vi "UHR-Fleezers Control (host) -TL - oscillation.vi"(0 "Tab Control":T5(tab)) -> ()   [LabVIEW 2013] (continued)
        n637 = property on="All Signals" class="WFChart (strict)"("Active Plot"=w1031) -> (error out=w1042:errorcluster)  [unwired: 2 in, 1 out]
        n638 = property on="All Signals" class="WFChart (strict)" props=["Plot", "Visible?", "Plot", "Plot Color"](error in=w1042) -> (error out=w1041:errorcluster, "Plot.Visible?"=w1040:bool)  [unwired: 1 in, 2 out]
        n639 = Select(t=FALSE ("Plot.Visible"), s=w1040, f=TRUE ("Plot.Visible")) -> (s? t:f=w1035:bool)
        n640 = property on="All Signals" class="WFChart (strict)"(error in=w1041, "Plot.Visible?"=w1035) -> (error out=w1037:errorcluster)  [unwired: 1 in, 1 out]
        n641 = property on="All Signals" class="WFChart (strict)"(error in=w1037) -> (error out=w1032:errorcluster, "Plot.Plot Color"=w1036:u32)  [unwired: 1 in, 1 out]
        n642 = property on="Signals to Plot" class="LstBox (strict)"(error in=w1032, "Active Row"=w1031) -> (error out=w1030:errorcluster)  [unwired: 1 in, 1 out]
        n643 = Select(t=w1036, s=w1035, f=u32 0) -> (s? t:f=w1033:u32)
        n644 = property on="Signals to Plot" class="LstBox (strict)"(error in=w1030, "CellFontColor"=w1033, "SelColor"=w1029, "CellBG"=w1029, "CellFontSize"=u32 20 ("Active Row:Cell Font:Size"), "CellFontBold"=TRUE ("Active Row:Cell Font:Bold")) -> ()  [unwired: 1 in, 2 out]
      }
      event "BD 1 Frequency 1 (MHz)", "BD 1 Frequency 2 (MHz)", "BD 1 Frequency 3 (MHz)", "BD 2 Frequency 1 (MHz)", "BD 2 Frequency 2 (MHz)", "BD 2 Frequency 3 (MHz)", "Trap Delta (MHz)": Value Change {
        # "anytime one of the frequencies is changed, write it to the RF board UNLESS Set 2 is being oscillated. The oscillation\nscript writes the frequencies to the RF board."
        n645 = event-data() -> ("CtlRef"=w1045:refnum<vi>)  [unwired: 6 out]
        n646 = control-ref of="Trap Delta (MHz)"() -> (w1044:refnum<vi>)
        n647 = Equal?(x=w1044, y=w1045) -> (x = y?=w1043:bool)
        n648 = case shown="False" "Oscillate Traps" {
          tunnel: w1048 -> [w1071 _]
          tunnel: [w1070 w1074] -> w1047
          tunnel: w1046 -> [w1069 w1074]
          tunnel: w1043 -> [w1056 _]
          frame False {
            w1050 = 80
            n649 = local read "BD 1 Frequency 2 (MHz)"() -> (w1058:dbl)
            n650 = Divide(x="Trap Delta (MHz)", y=2) -> (x/y=w1052:dbl)
            n651 = Subtract(x=w1050, y=w1052) -> (x-y=w1051:dbl)
            n652 = local write "BD 1 Frequency 1 (MHz)"(w1051) -> ()
            n653 = Add(x=w1050, y=w1052) -> (x+y=w1057:dbl)
            n654 = Select(t=w1057, s=w1056, f=w1058) -> (s? t:f=w1055:dbl)
            n655 = local read "Y RF Frequency Limits (MHz)"() -> (w1059:T16)
            n656 = local read "X RF Frequency Limits (MHz)"() -> (w1060:T16)
            n657 = local read "BD 1 Frequency 3 (MHz)"() -> (w1072:dbl)
            n658 = local write "BD 1 Frequency 2 (MHz)"(w1055) -> ()
            n659 = local read "BD 2 Frequency 1 (MHz)"() -> (w1063:dbl)
            n660 = local read "BD 2 Frequency 2 (MHz)"() -> (w1062:dbl)
            n661 = local read "BD 2 Frequency 3 (MHz)"() -> (w1073:dbl)
            n662 = call "set RF board frequency - interlace.vi"("Board 2 Frequency Limits"=w1059, "Board 1 Frequency Limits"=w1060, "error in"=w1069, "FPGA VI Reference In"=w1071, "Board 2 Frequency 3 (MHz)"=w1073, "Board 1 Frequency 3 (MHz)"=w1072, "Board 2 Frequency 2 (MHz)"=w1062, "Board 2 Frequency 1 (MHz)"=w1063, "Board 1 Frequency 2 (MHz)"=w1055, "Board 1 Frequency 1  (MHz)"=w1051) -> ("error out"=w1070:errorcluster)  [unwired: 1 out]
            n663 = Subtract(x=w1063, y=w1062) -> (x-y=w1067:dbl)
            n664 = Subtract(x=w1055, y=w1051) -> (x-y=w1068:dbl)
            n665 = Square(x=w1067) -> (x^2=w1065:dbl)
            n666 = Square(x=w1068) -> (x^2=w1066:dbl)
            n667 = Add(x=w1066, y=w1065) -> (x+y=w1064:dbl)
            n668 = Square Root(x=w1064) -> (sqrt(x)=w1061:dbl)
            n669 = local write "Trap Delta (MHz)"(w1061) -> ()
            n670 = property on="Initial delta (MHz)" class="DigNum (strict)"("Val(Sgnl)"=w1061) -> ()  [unwired: 2 in, 2 out]
          }
          frame True {
          }
        }
      }
      event "Round T1 X": Value Change {
        n671 = event-data() -> ()  [unwired: 7 out]
        n672 = local read "BD 1 Frequency 1 (MHz)"() -> (w1077:dbl)
        n673 = Round To Nearest(number=w1077) -> (nearest integer value=w1076:dbl)
        n674 = property on="BD 1 Frequency 1 (MHz)" class="DigNum (strict)"("Val(Sgnl)"=w1076) -> ()  [unwired: 2 in, 2 out]
      }
      event "Restart RF": Value Change {
        n675 = event-data() -> ()  [unwired: 7 out]
        n676 = xnode "Read/Write Control"("FPGA VI Reference In"=w1115, "error in"=w1110, "FPGA Controls  RF Box"=FALSE) -> ("FPGA VI Reference Out"=w1114:T19, "error out"=w1109:errorcluster)
        n677 = local read "Y RF Amplitude Limits (%)"() -> (w1090:T16)
        n678 = local read "X RF Amplitude Limits (%)"() -> (w1091:T16)
        n679 = local read "X RF Frequency Limits (MHz)"() -> (w1093:T16)
        n680 = local read "Y RF Frequency Limits (MHz)"() -> (w1092:T16)
        n681 = xnode "Read/Write Control"("FPGA VI Reference In"=w1114, "error in"=w1109, "Direct RF Box  Communication"=TRUE) -> ("FPGA VI Reference Out"=w1113:T19, "error out"=w1108:errorcluster)
        n682 = local read "BD 2 Frequency 3 (MHz)"() -> (w1100:dbl)
        n683 = local read "BD 2 Frequency 2 (MHz)"() -> (w1101:dbl)
        n684 = local read "BD 1 Frequency 3 (MHz)"() -> (w1104:dbl)
        n685 = local read "BD 1 Frequency 1 (MHz)"() -> (w1105:dbl)
        n686 = local read "BD 2 Frequency 1 (MHz)"() -> (w1102:dbl)
        n687 = local read "BD 1 Frequency 2 (MHz)"() -> (w1103:dbl)
        n688 = call "Initialize RF boards - interlace 3.vi"("error in"=w1108, "FPGA VI Reference In"=w1113) -> ("error out"=w1107:errorcluster, "FPGA VI Reference Out"=w1112:T19)
        n689 = local read "BD 2 Amplitude 2 (%)"() -> (w1095:dbl)
        n690 = local read "BD 2 Amplitude 1 (%)"() -> (w1096:dbl)
        n691 = local read "BD 2 Amplitude 3 (%)"() -> (w1094:dbl)
        n692 = local read "BD 1 Amplitude 3 (%)"() -> (w1099:dbl)
        n693 = local read "BD 1 Amplitude 1 (%)"() -> (w1098:dbl)
        n694 = local read "BD 1 Amplitude 2 (%)"() -> (w1097:dbl)
        n695 = call "set RF board frequency - interlace.vi"("Board 2 Frequency Limits"=w1092, "Board 1 Frequency Limits"=w1093, "error in"=w1107, "FPGA VI Reference In"=w1112, "Board 2 Frequency 3 (MHz)"=w1100, "Board 1 Frequency 3 (MHz)"=w1104, "Board 2 Frequency 2 (MHz)"=w1101, "Board 2 Frequency 1 (MHz)"=w1102, "Board 1 Frequency 2 (MHz)"=w1103, "Board 1 Frequency 1  (MHz)"=w1105) -> ("error out"=w1106:errorcluster, "FPGA VI Reference Out"=w1111:T19)
        n696 = call "set RF board amplitude - interlace.vi"("Board 2 Amplitude Limits"=w1090, "Board 1 Amplitude Limits"=w1091, "error in"=w1106, "FPGA VI Reference In"=w1111, "Board 2 Amplitude 3 (%)"=w1094, "Board 1 Amplitude 3 (%)"=w1099, "Board 2 Amplitude 2 (%)"=w1095, "Board 2 Amplitude 1 (%)"=w1096, "Board 1 Amplitude 2 (%)"=w1097, "Board 1 Amplitude 1 (%)"=w1098) -> ("error out"=w1083:errorcluster, "FPGA VI Reference Out"=w1087:T19)
        n697 = xnode "Read/Write Control"("FPGA VI Reference In"=w1087, "error in"=w1083, "Direct RF Box  Communication"=FALSE) -> ("FPGA VI Reference Out"=w1086:T19, "error out"=w1085:errorcluster)
        n698 = flat-sequence {
          tunnel: w1085 -> [w1116]
          tunnel: [w1116] -> w1084
          frame #0 {
            n699 = Wait (ms)(milliseconds to wait=u32 50) -> ()  [unwired: 1 out]
          }
        }
        n700 = xnode "Read/Write Control"("FPGA VI Reference In"=w1086, "error in"=w1084, "FPGA Controls  RF Box"=TRUE) -> ("error out"=w1079:errorcluster)  [unwired: 1 out]
        n701 = property on="Restart RF" class="Bool (strict)"(error in=w1079, "Value"=FALSE ("Restart RF")) -> (error out=w1078:errorcluster)  [unwired: 1 in, 1 out]
      }
      event "Round T2 X": Value Change {
        n702 = event-data() -> ()  [unwired: 7 out]
        n703 = local read "BD 1 Frequency 2 (MHz)"() -> (w1119:dbl)
        n704 = Round To Nearest(number=w1119) -> (nearest integer value=w1118:dbl)
        n705 = property on="BD 1 Frequency 2 (MHz)" class="DigNum (strict)"("Val(Sgnl)"=w1118) -> ()  [unwired: 2 in, 2 out]
      }
      event "Stop All": Value Change {
        n706 = event-data() -> ()  [unwired: 7 out]
        n707 = call "hamilton_controller.vi"("action"=T20."DISCONNECT") -> ()  [unwired: 10 in, 1 out]
        n708 = local read "Stop All"() -> (w1122:bool)
      }
      event "Delayed Interlace Start": Value Change {
        n709 = event-data() -> ()  [unwired: 7 out]
        n710 = flat-sequence {
          frame #0 {
            n711 = Multiply(x="Delay to Interlace (s)", y=1000.0) -> (x*y=w1125:dbl)
            n712 = Wait (ms)(milliseconds to wait=w1125) -> ()  [unwired: 1 out]
          }
          frame #1 {
            n713 = property on="Green laser mode" class="RadioBtnsControl (strict)"("Val(Sgnl)"=enum32{"Laser ON", "Laser OFF", "Interlace"}."Interlace" ("Value (Signaling)")) -> ()  [unwired: 2 in, 2 out]
          }
        }
      }
      event "BD 1 Amplitude 1 (%)", "BD 1 Amplitude 2 (%)", "BD 1 Amplitude 3 (%)", "BD 2 Amplitude 1 (%)", "BD 2 Amplitude 2 (%)", "BD 2 Amplitude 3 (%)", "Trap 1 ON", "Trap 2 ON", "Trap 3 ON", "Feedback On/Off", "All FB On/Off": Value Change {
        w1149 = i16 1 ("f")
        n714 = event-data() -> ()  [unwired: 7 out]
        n715 = local write "Trap 1 (ON/OFF)"("Trap 1 ON") -> ()
        n716 = local write "Trap 2 (ON/OFF)"("Trap 2 ON") -> ()
        n717 = Boolean To (0,1)(Boolean="Trap 3 ON") -> (0, 1=w1150:i16)
        n718 = Boolean To (0,1)(Boolean="Trap 1 ON") -> (0, 1=w1151:i16)
        n719 = Boolean To (0,1)(Boolean="Trap 2 ON") -> (0, 1=w1152:i16)
        n720 = Select(t=w1152, s="Trap ON/OFF X or Y Amp?", f=w1149) -> (s? t:f=w1147:i16)
        n721 = Select(t=w1151, s="Trap ON/OFF X or Y Amp?", f=w1149) -> (s? t:f=w1148:i16)
        n722 = Select(t=w1150, s="Trap ON/OFF X or Y Amp?", f=w1149) -> (s? t:f=w1146:i16)
        n723 = Select(t=w1149, s="Trap ON/OFF X or Y Amp?", f=w1152) -> (s? t:f=w1144:i16)
        n724 = Select(t=w1149, s="Trap ON/OFF X or Y Amp?", f=w1151) -> (s? t:f=w1145:i16)
        n725 = Select(t=w1149, s="Trap ON/OFF X or Y Amp?", f=w1150) -> (s? t:f=w1143:i16)
        n726 = And(x="All FB On/Off", y="Feedback On/Off") -> (x .and. y?=w1141:cluster{"Set 1":bool, "Set 2":bool})
        n727 = local read "BD 1 Amplitude 1 (%)"() -> (w1161:dbl)
        n728 = local read "BD 1 Amplitude 2 (%)"() -> (w1160:dbl)
        n729 = local read "BD 1 Amplitude 3 (%)"() -> (w1159:dbl)
        n730 = Unbundle By Name(w1141) -> ("Set 1"=w1136:bool, "Set 2"=w1133:bool)
        n731 = local read "Y RF Amplitude Limits (%)"() -> (w1129:T16)
        n732 = local read "X RF Amplitude Limits (%)"() -> (w1130:T16)
        n733 = local read "BD 2 Amplitude 1 (%)"() -> (w1162:dbl)
        n734 = local read "BD 2 Amplitude 2 (%)"() -> (w1163:dbl)
        n735 = local read "BD 2 Amplitude 3 (%)"() -> (w1164:dbl)
        n736 = And(x="Trap 2 ON", y=w1133) -> (x .and. y?=w1131:bool)
        n737 = And(x="Trap 1 ON", y=w1136) -> (x .and. y?=w1134:bool)
        n738 = Multiply(x=w1148, y=w1161) -> (x*y=w1156:dbl)
        n739 = Multiply(x=w1160, y=w1147) -> (x*y=w1154:dbl)
        n740 = Multiply(x=w1159, y=w1146) -> (x*y=w1155:dbl)
        n741 = Multiply(x=w1162, y=w1145) -> (x*y=w1165:dbl)
        n742 = Multiply(x=w1163, y=w1144) -> (x*y=w1166:dbl)
        n743 = Multiply(x=w1164, y=w1143) -> (x*y=w1167:dbl)
        n744 = call "set RF board amplitude - interlace.vi"("Board 2 Amplitude Limits"=w1129, "Board 1 Amplitude Limits"=w1130, "error in"=w1157, "FPGA VI Reference In"=w1158, "Board 2 Amplitude 3 (%)"=w1167, "Board 1 Amplitude 3 (%)"=w1155, "Board 2 Amplitude 2 (%)"=w1166, "Board 2 Amplitude 1 (%)"=w1165, "Board 1 Amplitude 2 (%)"=w1154, "Board 1 Amplitude 1 (%)"=w1156) -> ("error out"=w1138:errorcluster, "FPGA VI Reference Out"=w1139:T19)
        n745 = xnode "Read/Write Control"("FPGA VI Reference In"=w1139, "error in"=w1138, "FB On/Off Set 1"=w1134, "FB On/Off Set 2"=w1131) -> ("error out"=w1137:errorcluster)  [unwired: 1 out]
      }
      event "Load parameters": Value Change {
        n746 = event-data() -> ()  [unwired: 7 out]
        n747 = property on="Saved AOD Raster Scan Parameter Sets" class="Arr (strict)"() -> ("Index Values"=w1178:u32[])  [unwired: 2 in, 2 out]
        n748 = Index Array(array=w1178, index=0) -> (element=w1175:u32)
        n749 = local write "Load parameters"(FALSE ("Load parameters")) -> ()
        n750 = Index Array(array="Saved AOD Raster Scan Parameter Sets", index=w1175) -> (element=w1174:T30)
        n751 = Unbundle By Name(w1174) -> ("Scan Range AOD (nm) 2"=w1173:dbl, "Step Size AOD (nm) 2"=w1172:dbl, "Scan Speed AOD (nm/s) 2"=w1171:dbl, "Number of scans (AOD) 2"=w1170:u16)
        n752 = flat-sequence {
          tunnel: w1173 -> [w1181]
          tunnel: w1172 -> [w1180]
          tunnel: w1171 -> [w1179]
          tunnel: w1170 -> [w1182]
          frame #0 {
            n753 = local write "Scan Speed (nm/s)"(w1179) -> ()
            n754 = local write "Scan Range (nm)"(w1181) -> ()
            n755 = local write "Step Size (nm)"(w1180) -> ()
          }
          frame #1 {
            n756 = property on="Number of F/B Scans (AOD)" class="DigNum (strict)"("Val(Sgnl)"=w1182) -> ()  [unwired: 2 in, 2 out]
          }
        }
      }
      event "Trap 1 (ON/OFF)", "Trap 2 (ON/OFF)": Value Change {
        n757 = event-data() -> ()  [unwired: 7 out]
        n758 = property on="Trap 2 ON" class="Bool (strict)"("Val(Sgnl)"="Trap 2 (ON/OFF)") -> ()  [unwired: 2 in, 2 out]
        n759 = property on="Trap 1 ON" class="Bool (strict)"("Val(Sgnl)"="Trap 1 (ON/OFF)") -> ()  [unwired: 2 in, 2 out]
      }
      event "DIO count 1 (ticks)", "DIO count 2 (ticks)", "DIO count 3 (ticks)", "Interlace", "Number Interlace Sets", "Not-Interlacing Set": Value Change {
        n760 = event-data() -> ()  [unwired: 7 out]
        n761 = local read "DIO count 3 (ticks)"() -> (w1195:u32)
        n762 = local read "DIO count 1 (ticks)"() -> (w1197:u32)
        n763 = local read "DIO count 2 (ticks)"() -> (w1196:u32)
        n764 = To Unsigned Byte Integer(number="Not-Interlacing Set") -> (unsigned 8bit integer=w1186:u8)
        n765 = Add(x=w1186, y=u8 1) -> (x+y=w1190:u8)
        n766 = xnode "Read/Write Control"("FPGA VI Reference In"=w1201, "error in"=w1199, "DIO count 1 (ticks)"=w1197, "DIO count 2 (ticks)"=w1196, "DIO count 3 (ticks)"=w1195, "Interlace ON/OFF"="Interlace", "Number Interlace Cycles"="Number Interlace Sets", "Interlace Off Parameters"=w1190) -> ("error out"=w1200:errorcluster)  [unwired: 1 out]
        n767 = Build Array(w1197, w1196, w1195) -> (w1188:u32[])
        n768 = Split 1D Array(array=w1188, index="Number Interlace Sets") -> (first subarray=w1198:u32[])  [unwired: 1 out]
        n769 = Index Array(array=w1188, index=w1186) -> (element=w1187:u32)
        n770 = Add Array Elements(numeric array=w1198) -> (sum=w1192:u32)
        n771 = Select(t=w1192, s="Interlace", f=w1187) -> (s? t:f=→"Total Counts (ticks)":u32)
      }
      event "Reset Feedback": Value Change {
        n772 = event-data() -> ()  [unwired: 7 out]
        n773 = Unbundle By Name("Reset Feedback") -> ("Set 1"=w1205:bool, "Set 2"=w1204:bool)
        n774 = xnode "Read/Write Control"("FPGA VI Reference In"=w1207, "error in"=w1202, "FB Reset Set 1"=w1205, "FB Reset Set 2"=w1204) -> ("error out"=w1203:errorcluster)  [unwired: 1 out]
      }
      event "PID Gains": Value Change {
        n775 = event-data() -> ()  [unwired: 7 out]
        n776 = Unbundle By Name("PID Gains") -> ("Set 1"=w1211:T14, "Set 2"=w1210:T14)
        n777 = xnode "Read/Write Control"("FPGA VI Reference In"=w1212, "error in"=w1208, "FB Gains Set 1"=w1211, "FB Gains Set 2"=w1210) -> ("error out"=w1209:errorcluster)  [unwired: 1 out]
      }
      event "AI2 to Setpoint", "Trap Intensity\nSetpoints (V)": Value Change {
        n778 = event-data() -> ()  [unwired: 7 out]
        n779 = xnode "Read/Write Control"("FPGA VI Reference In"=w1218, "error in"=w1214) -> ("FPGA VI Reference Out"=w1217:T19, "error out"=w1216:errorcluster, "AI2 Y Sum Set 1"=w1225:i16, "AI2 Y Sum Set 2"=w1224:i16)
        n780 = Cluster To Array(cluster="AI2 to Setpoint") -> (array=w1228:bool[])
        n781 = local read "AI2 (V)"() -> (w1226:cluster{"Set 1":dbl, "Set 2":dbl})
        n782 = Or Array Elements(Boolean array=w1228) -> (logical OR=w1229:bool)
        n783 = Bundle By Name(cluster=w1226, "Set 1"=w1225, "Set 2"=w1224) -> (w1223:cluster{"Set 1":dbl, "Set 2":dbl})
        n784 = Divide(x=w1223, y=3276.7) -> (x/y=w1222:cluster{"Set 1":dbl, "Set 2":dbl})
        "AI2 (V)" <- w1222
        n785 = case shown="True" w1229 {
          tunnel: [w1232 w1249] -> w1221
          tunnel: "AI2 to Setpoint" -> [_ w1245]
          tunnel: "Trap Intensity\nSetpoints (V)" -> [w1233 w1248]
          tunnel: w1222 -> [_ w1242]
          frame False {
            n786 = Multiply(x=3276.7, y=w1233) -> (x*y=w1234:cluster{"Set 1":dbl, "Set 2":dbl})
            n787 = To Word Integer(number=w1234) -> (16bit integer=w1232:cluster{"Set 1":i16, "Set 2":i16})
          }
          frame True {
            n788 = Unbundle By Name(w1242) -> ("Set 1"=w1241:dbl, "Set 2"=w1240:dbl)
            n789 = Unbundle By Name(w1248) -> ("Set 1"=w1247:dbl, "Set 2"=w1246:dbl)
            n790 = Unbundle By Name(w1245) -> ("Set 1"=w1244:bool, "Set 2"=w1243:bool)
            n791 = Select(t=w1241, s=w1244, f=w1247) -> (s? t:f=w1239:dbl)
            n792 = Select(t=w1240, s=w1243, f=w1246) -> (s? t:f=w1238:dbl)
            n793 = Bundle By Name(cluster=w1248, "Set 1"=w1239, "Set 2"=w1238) -> (w1236:cluster{"Set 1":dbl, "Set 2":dbl})
            n794 = local write "Trap Intensity\nSetpoints (V)"(w1236) -> ()
            n795 = Multiply(x=3276.7, y=w1236) -> (x*y=w1237:cluster{"Set 1":dbl, "Set 2":dbl})
            n796 = To Word Integer(number=w1237) -> (16bit integer=w1249:cluster{"Set 1":i16, "Set 2":i16})
          }
        }
        n797 = Unbundle By Name(w1221) -> ("Set 1"=w1220:i16, "Set 2"=w1219:i16)
        n798 = xnode "Read/Write Control"("FPGA VI Reference In"=w1217, "error in"=w1216, "FB Setpoint Set 1"=w1220, "FB Setpoint Set 2"=w1219) -> ("error out"=w1215:errorcluster)  [unwired: 1 out]
      }
      event "Invert GI": Value Change {
        n799 = event-data() -> ()  [unwired: 7 out]
        n800 = xnode "Read/Write Control"("FPGA VI Reference In"=w1254, "error in"=w1252, "Invert GI"="Invert GI", "Invert GI 2"="Invert GI") -> ("error out"=w1253:errorcluster)  [unwired: 1 out]
      }
      event "Green FB Setpoint (mV)", "Green FB Gains", "Green FB On/Off", "Current When FB OFF (%)", "Green int current ON count adj": Value Change {
        n801 = event-data() -> ()  [unwired: 7 out]
        n802 = local read "Green FB Setpoint (mV)"() -> (w1261:dbl)
        n803 = local read "Current When FB OFF (%)"() -> (w1264:dbl)
        n804 = Multiply(x=w1261, y=3.2767) -> (x*y=w1260:dbl)
        n805 = Multiply(x=w1264, y=655.35) -> (x*y=w1265:dbl)
        n806 = To Unsigned Word Integer(number=w1265) -> (unsigned 16bit integer=w1263:u16)
        n807 = local read "Green int current ON count adj"() -> (w1268:u32)
        n808 = local read "Green FB Gains"() -> (w1267:T14)
        n809 = local read "Green Laser ON/Interlacing"() -> (w1258:bool)
        n810 = local read "Green laser mode"() -> (w1257:enum32{"Laser ON", "Laser OFF", "Interlace"})
        n811 = local read "Green FB On/Off"() -> (w1269:bool)
        n812 = Equal?(x=w1257, y=enum32{"Laser ON", "Laser OFF", "Interlace"}."Interlace") -> (x = y?=w1255:bool)
        n813 = Compound Arithmetic op=AND(w1255, w1269, w1258) -> (w1259:bool)
        n814 = xnode "Read/Write Control"("FPGA VI Reference In"=w1272, "error in"=w1271, "Green FB Setpoint"=w1260, "Green FB On/Off"=w1259, "Current Out"=w1263, "Green int current ON count adj"=w1268, "Green FB Gains"=w1267) -> ("error out"=w1270:errorcluster)  [unwired: 1 out]
      }
      event "Green laser mode", "Green Laser ON/Interlacing": Value Change {
        n815 = event-data() -> ()  [unwired: 7 out]
        n816 = case shown="True" "Green Laser ON/Interlacing" {
          tunnel: "Green laser mode" -> [_ w1286]
          tunnel: [enum32{"Laser ON", "Laser OFF", "Interlace"}."Laser OFF" ("Green laser mode") w1286] -> w1274
          tunnel: [FALSE w1282] -> w1273
          frame False {
          }
          frame True {
            n817 = local read "Green FB On/Off"() -> (w1283:bool)
            n818 = Equal?(x=w1286, y=enum32{"Laser ON", "Laser OFF", "Interlace"}."Interlace") -> (x = y?=w1284:bool)
            n819 = And(x=w1284, y=w1283) -> (x .and. y?=w1282:bool)
          }
        }
        n820 = xnode "Read/Write Control"("FPGA VI Reference In"=w1279, "error in"=w1277, "Operating Mode"=w1274, "Operating Mode 2"=w1274, "Green FB On/Off"=w1273) -> ("error out"=w1278:errorcluster)  [unwired: 1 out]
      }
      event "- phase (APD 1 Gate)", "+ phase (APD 1 Gate)": Value Change {
        n821 = event-data() -> ()  [unwired: 7 out]
        n822 = local read "Phase Adj. (APD 1 Gate)"() -> (w1287:i16)
        n823 = Negate(x=w1287) -> (-x=w1295:i16)
        n824 = Select(t=w1295, s="- phase (APD 1 Gate)", f=w1287) -> (s? t:f=w1294:i16)
        n825 = Or(x="- phase (APD 1 Gate)", y="+ phase (APD 1 Gate)") -> (x .or. y?=w1290:bool)
        n826 = xnode "Read/Write Control"("FPGA VI Reference In"=w1297, "error in"=w1296, "Phase count adjustment (APD 1 Gate)"=w1294) -> ("FPGA VI Reference Out"=w1292:T19, "error out"=w1293:errorcluster)
        n827 = xnode "Read/Write Control"("FPGA VI Reference In"=w1292, "error in"=w1293, "+ phase (APD 1 Gate)"=w1290) -> ("error out"=w1291:errorcluster)  [unwired: 1 out]
      }
      event "+ phase (APD 2 Gate)", "- phase (APD 2 Gate)": Value Change {
        n828 = event-data() -> ()  [unwired: 7 out]
        n829 = local read "Phase Adj. (APD 2 Gate)"() -> (w1298:i16)
        n830 = Negate(x=w1298) -> (-x=w1306:i16)
        n831 = Select(t=w1306, s="- phase (APD 2 Gate)", f=w1298) -> (s? t:f=w1305:i16)
        n832 = Or(x="- phase (APD 2 Gate)", y="+ phase (APD 2 Gate)") -> (x .or. y?=w1301:bool)
        n833 = xnode "Read/Write Control"("FPGA VI Reference In"=w1308, "error in"=w1307, "Phase count adjustment (APD 2 Gate)"=w1305) -> ("FPGA VI Reference Out"=w1303:T19, "error out"=w1304:errorcluster)
        n834 = xnode "Read/Write Control"("FPGA VI Reference In"=w1303, "error in"=w1304, "+ phase (APD 2 Gate)"=w1301) -> ("error out"=w1302:errorcluster)  [unwired: 1 out]
      }
      event "Phase Adj. (APD Acq)", "+ phase (APD Acq)", "- phase (APD Acq)": Value Change {
        n835 = event-data() -> ()  [unwired: 7 out]
        n836 = local read "Phase Adj. (APD Acq)"() -> (w1311:i16)
        n837 = Negate(x=w1311) -> (-x=w1317:i16)
        n838 = Select(t=w1317, s="+ phase (APD Acq)", f=w1311) -> (s? t:f=w1316:i16)
        n839 = Or(x="+ phase (APD Acq)", y="- phase (APD Acq)") -> (x .or. y?=w1312:bool)
        n840 = xnode "Read/Write Control"("FPGA VI Reference In"=w1319, "error in"=w1318, "Phase Count Adjustment (APD Acq)"=w1316) -> ("FPGA VI Reference Out"=w1314:T19, "error out"=w1315:errorcluster)
        n841 = xnode "Read/Write Control"("FPGA VI Reference In"=w1314, "error in"=w1315, "+ phase (APD Acq)"=w1312) -> ("error out"=w1313:errorcluster)  [unwired: 1 out]
      }
      event "Phase adj. (GI)", "+ phase (GI)", "- phase (GI)": Value Change {
        n842 = event-data() -> ()  [unwired: 7 out]
        n843 = Negate(x="Phase adj. (GI)") -> (-x=w1328:i16)
        n844 = Select(t=w1328, s="+ phase (GI)", f="Phase adj. (GI)") -> (s? t:f=w1327:i16)
        n845 = Or(x="+ phase (GI)", y="- phase (GI)") -> (x .or. y?=w1323:bool)
        n846 = xnode "Read/Write Control"("FPGA VI Reference In"=w1330, "error in"=w1329, "Phase count adjustment (GI)"=w1327) -> ("FPGA VI Reference Out"=w1325:T19, "error out"=w1326:errorcluster)
        n847 = xnode "Read/Write Control"("FPGA VI Reference In"=w1325, "error in"=w1326, "+ phase (GI)"=w1323) -> ("error out"=w1324:errorcluster)  [unwired: 1 out]
      }
      event "Phase adj. (GI) 2", "+ phase (GI) 2", "- phase (GI) 2": Value Change {
        n848 = event-data() -> ()  [unwired: 7 out]
        n849 = Negate(x="Phase adj. (GI) 2") -> (-x=w1339:i16)
        n850 = Select(t=w1339, s="+ phase (GI) 2", f="Phase adj. (GI) 2") -> (s? t:f=w1338:i16)
        n851 = Or(x="+ phase (GI) 2", y="- phase (GI) 2") -> (x .or. y?=w1334:bool)
        n852 = xnode "Read/Write Control"("FPGA VI Reference In"=w1341, "error in"=w1340, "Phase count adjustment (GI) 2"=w1338) -> ("FPGA VI Reference Out"=w1336:T19, "error out"=w1337:errorcluster)
        n853 = xnode "Read/Write Control"("FPGA VI Reference In"=w1336, "error in"=w1337, "+ phase (GI) 2"=w1334) -> ("error out"=w1335:errorcluster)  [unwired: 1 out]
      }
      event "Phase adj. (Green FB)", "- phase (Green FB)", "+ phase (Green FB)": Value Change {
        n854 = event-data() -> ()  [unwired: 7 out]
        n855 = Negate(x="Phase adj. (Green FB)") -> (-x=w1350:i16)
        n856 = Select(t=w1350, s="+ phase (Green FB)", f="Phase adj. (Green FB)") -> (s? t:f=w1349:i16)
        n857 = Or(x="+ phase (Green FB)", y="- phase (Green FB)") -> (x .or. y?=w1345:bool)
        n858 = xnode "Read/Write Control"("FPGA VI Reference In"=w1352, "error in"=w1351, "Phase count adjustment (Green FB)"=w1349) -> ("FPGA VI Reference Out"=w1347:T19, "error out"=w1348:errorcluster)
        n859 = xnode "Read/Write Control"("FPGA VI Reference In"=w1347, "error in"=w1348, "+ phase (Green FB)"=w1345) -> ("error out"=w1346:errorcluster)  [unwired: 1 out]
      }
      event "Invert APD Gate", "APD Gate ON Count", "APD Gate OFF Count", "APD Gate", "APD Integration Time (s)", "APD 1 AO Mult.", "APD 2 AO Mult.": Value Change {
        n860 = event-data() -> ()  [unwired: 7 out]
        n861 = local read "APD Integration Time (s)"() -> (w1353:dbl)
        n862 = local read "APD Gate ON Count"() -> (w1366:u32)
        n863 = local read "APD Gate OFF Count"() -> (w1365:u32)
        n864 = local read "Invert APD Gate"() -> (w1367:bool)
        n865 = local read "APD Gate"() -> (w1364:enum32{"ON", "OFF", "Interlace"})
        n866 = Multiply(x=w1353, y=40000000.0) -> (x*y=w1362:dbl)
        n867 = Reciprocal(x=w1353) -> (1/x=→"APD Acq Rate (Hz)":dbl)
        n868 = To Unsigned Long Integer(number=w1362) -> (unsigned 32bit integer=w1361:u32)
        n869 = local read "DMA Update Period (s)"() -> (w1354:dbl)
        n870 = Divide(x=w1354, y=w1353) -> (x/y=w1357:dbl)
        n871 = local read "APD 1 AO Mult."() -> (w1359:i16)
        n872 = local read "APD 2 AO Mult."() -> (w1358:i16)
        n873 = Multiply(x=2.0, y=w1357) -> (x*y=w1356:dbl)
        n874 = local write "APD Samples/FIFO Acq."(w1357) -> ()
        n875 = local write "APD Elements/DMA read"(w1356) -> ()
        n876 = xnode "Read/Write Control"("FPGA VI Reference In"=w1370, "error in"=w1369, "Invert APD Gate"=w1367, "APD Gate ON Count"=w1366, "APD Gate OFF Count"=w1365, "APD Acq Rate Count"=w1361, "APD Gate Operating Mode"=w1364, "APD 1 AO scale factor"=w1359, "APD 2 AO scale factor"=w1358) -> ("error out"=w1368:errorcluster)  [unwired: 1 out]
      }
      event "GI Frequency, ON count", "Green FB Count", "GI Frequency, OFF count": Value Change {
        n877 = event-data() -> ()  [unwired: 7 out]
        n878 = xnode "Read/Write Control"("FPGA VI Reference In"=w1376, "error in"=w1374, "Green interlace ON count"="GI Frequency, ON count", "Green interlace OFF count"="GI Frequency, OFF count", "Green interlace ON count 2"="GI Frequency, ON count", "Green interlace OFF count 2"="GI Frequency, OFF count", "Green FB Count"="Green FB Count") -> ("error out"=w1375:errorcluster)  [unwired: 1 out]
      }
      event "Number of F/B Scans (AOD)", "Scan Speed (nm/s)", "Scan BD", "Initial delta (MHz)", "Step Size (nm)", "Scan Range (nm)": Value Change {
        w1438 = 123.0  # AOM cal (nm/MHz)
        n879 = event-data() -> ()  [unwired: 7 out]
        n880 = local read "BD 1 Frequency 1 (MHz)"() -> (w1421:dbl)
        n881 = local read "AOM X Cal (nm/MHz)"() -> (w1413:dbl)
        n882 = local read "X RF Frequency Limits (MHz)"() -> (w1425:T16)
        n883 = local read "Y RF Frequency Limits (MHz)"() -> (w1422:T16)
        n884 = local read "BD 2 Frequency 1 (MHz)"() -> (w1427:dbl)
        n885 = Negate(x="Scan Range (nm)") -> (-x=w1391:dbl)
        n886 = Divide(x=w1391, y=w1413) -> (x/y=w1395:dbl)
        n887 = Select(t=w1425, s="Scan BD", f=w1422) -> (s? t:f=w1424:T16)
        n888 = Select(t=w1421, s="Scan BD", f=w1427) -> (s? t:f=w1426:dbl)
        n889 = Unbundle By Name(w1424) -> ("Maximum"=w1433:dbl, "Minimum"=w1432:dbl)
        n890 = Add(x=w1395, y=w1426) -> (x+y=w1430:dbl)
        n891 = Divide(x=w1391, y="Step Size (nm)") -> (x/y=w1410:dbl)
        n892 = Divide(x="Step Size (nm)", y=w1413) -> (x/y=w1419:dbl)
        n893 = Absolute Value(x=w1410) -> (abs(x)=w1394:dbl)
        n894 = Sign(1:w1391) -> (0:w1392:dbl)
        n895 = In Range and Coerce(upper limit=w1433, x=w1430, lower limit=w1432) -> (coerced(x)=w1429:dbl, In Range?=w1431:bool)
        n896 = To Unsigned Quad Integer(1:w1394) -> (0:w1409:u64)
        "Scan steps (AOD)" <- w1409
        n897 = call "IR AOM freq to word.vi"("Frequency In (MHz)"=w1419) -> ("Frequency Word Out (double)"=w1416:dbl)
        n898 = Multiply(x=w1392, y=w1416) -> (x*y=w1393:dbl)
        n899 = Subtract(x=w1430, y=w1429) -> (x-y=w1428:dbl)
        n900 = To Quad Integer(1:w1393) -> (0:w1415:i64)
        "Incr. int (AOD)" <- w1415
        n901 = Subtract(x=w1395, y=w1428) -> (x-y=w1414:dbl)
        "Scan Range (MHz)" <- w1414
        n902 = Select(t=w1395, s=w1431, f=w1414) -> (s? t:f=w1434:dbl)
        n903 = Multiply(x=w1414, y=w1413) -> (x*y=w1412:dbl)
        n904 = Decrement(x=w1409) -> (x-1=w1462:u64)
        n905 = Negate(x=w1412) -> (-x=w1408:dbl)
        n906 = local write "Scan Range (nm)"(w1408) -> ()
        n907 = Divide(x=w1434, y=w1462) -> (x/y=w1418:dbl)
        "Scan Increment (MHz)" <- w1418
        n908 = call "IR AOM freq to word.vi"("Frequency In (MHz)"=w1418) -> ("Frequency Word Out (double)"=w1417:dbl)
        n909 = Divide(x="Step Size (nm)", y="Scan Speed (nm/s)") -> (x/y=w1405:dbl)
        n910 = To Quad Integer(1:w1417) -> ()  [unwired: 1 out]
        n911 = local read "Number Interlace Sets"() -> (w1389:u8)
        n912 = local read "AI Count (ticks)"() -> (w1390:u32)
        n913 = local read "Total Counts (ticks)"() -> (w1388:u32)
        n914 = local read "# Samples/trap"() -> (w1420:u32)
        n915 = Multiply(x=w1390, y=w1389) -> (x*y=w1387:u32)
        n916 = Divide(x=w1388, y=w1387) -> (x/y=w1386:dbl)
        n917 = Select(t=w1421, s="Scan BD", f=w1427) -> (s? t:f=w1459:dbl)
        "Initial freq. (MHz)" <- w1459
        n918 = Add(x=w1434, y=w1459) -> (x+y=→"Final freq. (MHz)":dbl)
        n919 = Divide(x=w1388, y=40000000.0) -> (x/y=w1404:dbl)
        n920 = Divide(x=w1405, y=w1404) -> (x/y=w1403:dbl)
        n921 = To Unsigned Quad Integer(1:w1403) -> (0:w1378:u64)
        n922 = Quotient & Remainder(x=w1378, y=u64 2) -> (x-y*floor(x/y)=w1382:u64)  [unwired: 1 out]
        n923 = Equal?(x=w1382, y=u64 0) -> (x = y?=w1380:bool)
        n924 = Decrement(x=w1378) -> (x-1=w1379:u64)
        n925 = Select(t=w1378, s=w1380, f=w1379) -> (s? t:f=w1377:u64)
        "Cycles/step (AOD)" <- w1377
        n926 = xnode "Read/Write Control"("FPGA VI Reference In"=w1470, "error in"=w1469, "Scan steps"=w1409, "Number of scans"="Number of F/B Scans (AOD)", "Cycles per step"=w1377, "Scan freq.  increment"=w1415, "Scan BD"="Scan BD") -> ("error out"=w1468:errorcluster)  [unwired: 1 out]
        n927 = Multiply(x=w1409, y=w1377) -> (x*y=w1463:u64)
        n928 = Multiply(x=w1463, y=u64 2) -> (x*y=w1385:u64)
        n929 = Multiply(x=w1386, y=w1385) -> (x*y=w1384:dbl)
        "Data points/scan (f/b)" <- w1384
        n930 = Multiply(x=w1384, y="Number of F/B Scans (AOD)") -> (x*y=w1466:dbl)
        "Data points/scans" <- w1466
        n931 = Divide(x=w1466, y=w1420) -> (x/y=→"N sets should be saved":dbl)
        n932 = Multiply(x=w1463, y=w1404) -> (x*y=w1402:dbl)
        "Time/Scan (s) (AOD)" <- w1402
        n933 = Select(t=w1434, s="Scan BD", f=0.0) -> (s? t:f=w1460:dbl)
        n934 = Select(t=0.0, s="Scan BD", f=w1434) -> (s? t:f=w1456:dbl)
        n935 = local read "BD 2 Frequency 2 (MHz)"() -> (w1452:dbl)
        n936 = local read "BD 1 Frequency 2 (MHz)"() -> (w1455:dbl)
        n937 = Add(x=w1456, y=w1427) -> (x+y=w1453:dbl)
        n938 = Add(x=w1421, y=w1460) -> (x+y=w1454:dbl)
        n939 = Multiply(x=w1402, y=2.0) -> (x*y=w1401:dbl)
        n940 = Multiply(x=w1401, y="Number of F/B Scans (AOD)") -> (x*y=w1398:dbl)
        n941 = Divide(x=w1398, y=60.0) -> (x/y=→"Time to Finish All (min)":dbl)
        n942 = Add(x="Trap 2 Bead Size (nm)", y="Trap 1 Bead Size (nm)") -> (x+y=w1442:dbl)
        n943 = local read "Initial delta (MHz)"() -> (w1439:dbl)
        n944 = Divide(x=w1442, y=2.0) -> (x/y=w1436:dbl)
        n945 = Subtract(x=w1453, y=w1452) -> (x-y=w1450:dbl)
        n946 = Subtract(x=w1454, y=w1455) -> (x-y=w1451:dbl)
        n947 = Square(x=w1450) -> (x^2=w1449:dbl)
        n948 = Square(x=w1451) -> (x^2=w1448:dbl)
        n949 = Add(x=w1448, y=w1449) -> (x+y=w1447:dbl)
        n950 = Square Root(x=w1447) -> (sqrt(x)=w1446:dbl)
        "Final delta (MHz)" <- w1446
        n951 = Multiply(x=w1438, y=w1446) -> (x*y=w1445:dbl)
        n952 = Multiply(x=w1439, y=w1438) -> (x*y=w1437:dbl)
        n953 = Subtract(x=w1437, y=w1436) -> (x-y=→"Initial sep (nm)":dbl)
        n954 = Subtract(x=w1445, y=w1436) -> (x-y=→"Final sep (nm)":dbl)
      }
      event "Raster Scanning...": Value Change {
        n955 = event-data() -> ("NewVal"=w1471:bool)  [unwired: 6 out]
        n956 = case shown="True" w1471 {
          frame False {
          }
          frame True {
            n957 = property on="BD 1 Frequency 1 (MHz)" class="DigNum (strict)"("Val(Sgnl)"=65.0 ("Value (Signaling)")) -> ()  [unwired: 2 in, 2 out]
          }
        }
      }
      event "Freq or Amp switch first", "Swap F1 and F2", "Freq switch delay", "Amp switch delay": Value Change {
        n958 = event-data() -> ()  [unwired: 7 out]
        n959 = local read "Freq or Amp switch first"() -> (w1473:bool)
        n960 = local read "Amp switch delay"() -> (w1474:u16)
        n961 = local read "Freq switch delay"() -> (w1476:u16)
        n962 = local read "Swap F1 and F2"() -> (w1475:bool)
        n963 = xnode "Read/Write Control"("FPGA VI Reference In"=w1479, "error in"=w1478, "Freq switch delay"=w1476, "Swap F1 and F2"=w1475, "Amp switch delay"=w1474, "Freq or Amp switch first"=w1473) -> ("error out"=w1477:errorcluster)  [unwired: 1 out]
      }
      event "Scan steps (MCL)", "Number of scans (MCL)", "Scan Range (V)\n(of steps)", "2D or 1D Scan", "N APD Samp/step", "Fast Scan Dir", "Continuous MCL Scanning", "Scan lines (y)": Value Change {
        w1481 = 32767.0 ("y")
        n964 = event-data() -> ()  [unwired: 7 out]
        n965 = Select(t="Scan lines (y)", s="2D or 1D Scan", f="Number of scans (MCL)") -> (s? t:f=w1486:u64)
        n966 = Decrement(x="Scan steps (MCL)") -> (x-1=w1502:u64)
        n967 = Divide(x="Scan Range (V)\n(of steps)", y=w1502) -> (x/y=w1501:dbl)
        "Desired Scan Incr (V)" <- w1501
        n968 = local read "APD Integration Time (s)"() -> (w1494:dbl)
        n969 = Multiply(x=w1501, y=w1481) -> (x*y=w1510:dbl)
        n970 = Divide(x=w1510, y=10.0) -> (x/y=w1500:dbl)
        "Desired incr (int)" <- w1500
        n971 = local read "Update Count (MCL)"() -> (w1506:u32)
        n972 = Round Toward -Infinity(1:w1500) -> (0:w1509:dbl)
        n973 = To Word Integer(number=w1509) -> (16bit integer=w1484:i16)
        "Actual Incr. int (MCL)" <- w1484
        n974 = Multiply(x=w1494, y=40000000.0) -> (x*y=w1507:dbl)
        n975 = Divide(x=w1507, y=w1506) -> (x/y=w1505:dbl)
        n976 = Multiply(x=i16 10, y=w1484) -> (x*y=w1482:i16)
        n977 = Multiply(x="N APD Samp/step", y=w1505) -> (x*y=w1504:dbl)
        "Cycles/step (MCL)" <- w1504
        n978 = Divide(x=w1482, y=w1481) -> (x/y=→"Actual MCL Inc (V)":dbl)
        n979 = Multiply(x="N APD Samp/step", y="Scan steps (MCL)") -> (x*y=w1496:dbl)
        n980 = local read "APD Samples/FIFO Acq."() -> (w1493:dbl)
        n981 = Multiply(x=w1496, y=u64 2) -> (x*y=w1495:dbl)
        "Data points/scan (f+b)" <- w1495
        n982 = Multiply(x=w1495, y=w1486) -> (x*y=w1513:dbl)
        "Data points/scans (MCL)" <- w1513
        n983 = Multiply(x=w1494, y=w1495) -> (x*y=w1487:dbl)
        "Time/f+b scan (s) (MCL)" <- w1487
        n984 = Divide(x=w1513, y=w1493) -> (x/y=→"N sets should be saved (MCL)":dbl)
        n985 = Multiply(x=w1487, y=w1486) -> (x*y=→"Total Time (s)":dbl)
        n986 = Not(x="Fast Scan Dir") -> (.not. x?=w1491:bool)
        n987 = xnode "Read/Write Control"("FPGA VI Reference In"=w1517, "error in"=w1516, "Scan steps (MCL)"="Scan steps (MCL)", "Number of scans (MCL)"=w1486, "Cycles per step (MCL)"=w1504, "Scan freq.  increment (MCL)"=w1484, "1D or 2D Scan?"="2D or 1D Scan", "MCL Scan Axis"=w1491, "Cont. Scan (MCL)"="Continuous MCL Scanning") -> ("error out"=w1515:errorcluster)  [unwired: 1 out]
      }
      event "Read Cal": Value Change {
        w1521 = 1000.0 ("y")
        n988 = event-data() -> ()  [unwired: 7 out]
        n989 = local read "Save file name"() -> (w1544:path)
        n990 = local write "Read Cal"(FALSE ("Read Cal")) -> ()
        n991 = Strip Path(path=w1544) -> (stripped path=w1543:path)  [unwired: 1 out]
        n992 = Path To String(path=w1543) -> (string=w1542:string)
        n993 = Concatenate Strings(w1542, "\\current_oscill.cal" ("string")) -> (w1540:string)
        n994 = String To Path(string=w1540) -> (path=w1539:path)
        n995 = Open/Create/Replace File(file path (use dialog)=w1539, operation (0:open)=T23."open", access (0:read/write)=enum16{"read/write", "read-only", "write-only"}."read-only") -> (refnum out=w1547:refnum<file>, error out=w1533:errorcluster)  [unwired: 1 in, 3 out]
        n996 = Deny Access(4:w1533, 7:w1547) -> (0:w1532:errorcluster, 3:w1538:refnum<file>)  [unwired: 1 out]
        n997 = Read from Binary File(5:0.0, 8:w1532, 9:T29."big-endian, network order" ("byte order (0:big-endian, network order)"), 10:-1 ("count (1)"), 11:w1538) -> (0:w1531:errorcluster, 2:w1518:dbl[], 3:w1534:refnum<file>)  [unwired: 2 out]
        n998 = Array To Cluster(array=w1518) -> (cluster=w1519:T31)
        n999 = Unbundle(w1519) -> ("[0]"=w1529:dbl, "[1]"=w1528:dbl, "[2]"=w1527:dbl, "[3]"=w1526:dbl, "[4]"=w1525:dbl, "[5]"=w1524:dbl)
        n1000 = Close File(refnum=w1534, error in=w1531) -> (error out=→"Read cal error":errorcluster)  [unwired: 1 out]
        n1001 = Multiply(x=w1524, y=w1521) -> (x*y=w1522:dbl)
        n1002 = local write "T2 kappa_x (pN/nm)"(w1526) -> ()
        n1003 = local write "T1 kappa_x (pN/nm)"(w1527) -> ()
        n1004 = local write "T1 alpha_x (nm/V)"(w1529) -> ()
        n1005 = local write "T2 alpha_x (nm/V)"(w1528) -> ()
        n1006 = disable-structure shown="Disabled" {
          frame Disabled {
            n1007 = local read "Trap 2 Bead Size (nm)"() -> ()  [unwired: 1 in]
            n1008 = local read "Trap 1 Bead Size (nm)"() -> ()  [unwired: 1 in]
          }
          frame Enabled {
          }
        }
        n1009 = Multiply(x=w1525, y=w1521) -> (x*y=w1523:dbl)
        n1010 = local write "T1 offset_x (mV)"(w1523) -> ()
        n1011 = local write "T2 offset_x (mV)"(w1522) -> ()
      }
      event "Abort MCL Scan": Value Change {
        n1012 = event-data() -> ()  [unwired: 7 out]
        n1013 = local write "MCL Scanning"(FALSE ("MCL Scanning")) -> ()
        n1014 = xnode "Read/Write Control"("FPGA VI Reference In"=w1552, "error in"=w1551, "Abort scan (MCL)"="Abort MCL Scan") -> ("error out"=w1550:errorcluster)  [unwired: 1 out]
      }
      event "Update Count (MCL)": Value Change {
        n1015 = event-data() -> ()  [unwired: 7 out]
        n1016 = xnode "Read/Write Control"("FPGA VI Reference In"=w1556, "error in"=w1555, "MCL count"="Update Count (MCL)") -> ("error out"=w1554:errorcluster)  [unwired: 1 out]
      }
      event "Phase adjust (MCL)", "+ phase (MCL)", "- phase (MCL)": Value Change {
        n1017 = event-data() -> ()  [unwired: 7 out]
        n1018 = Negate(x="Phase adjust (MCL)") -> (-x=w1565:i16)
        n1019 = Select(t=w1565, s="- phase (MCL)", f="Phase adjust (MCL)") -> (s? t:f=w1563:i16)
        n1020 = Or(x="- phase (MCL)", y="+ phase (MCL)") -> (x .or. y?=w1558:bool)
        n1021 = xnode "Read/Write Control"("FPGA VI Reference In"=w1567, "error in"=w1566, "Phase count adjustment (MCL)"=w1563) -> ("FPGA VI Reference Out"=w1559:T19, "error out"=w1560:errorcluster)
        n1022 = xnode "Read/Write Control"("FPGA VI Reference In"=w1559, "error in"=w1560, "+ phase (MCL)"=w1558) -> ("error out"=w1557:errorcluster)  [unwired: 1 out]
      }
      event "Abort AOD Scan": Value Change {
        n1023 = event-data() -> ()  [unwired: 7 out]
        n1024 = xnode "Read/Write Control"("FPGA VI Reference In"=w1571, "error in"=w1570, "Abort scan"="Abort AOD Scan") -> ("error out"=w1569:errorcluster)  [unwired: 1 out]
      }
      event "Continuous AOD Scanning": Value Change {
        n1025 = event-data() -> ()  [unwired: 7 out]
        n1026 = xnode "Read/Write Control"("FPGA VI Reference In"=w1575, "error in"=w1574, "Cont. Scan"="Continuous AOD Scanning") -> ("error out"=w1573:errorcluster)  [unwired: 1 out]
      }
      event "Index": Value Change {
        n1027 = event-data() -> ()  [unwired: 7 out]
        n1028 = call "Create new save file.vi"("Insert"="", "Ext"=".dat" ("string"), "Index In"="Index") -> ("Path Out"=→"Save file name":path, "Index Out"=w1576:dbl)
        "Save index" <- w1576
        n1029 = local write "Index"(w1576) -> ()
      }
      event "AO1", "AO2": Value Change {
        w1591 = 10.0 ("y")
        w1590 = 32767.0 ("y")
        n1030 = event-data() -> ()  [unwired: 7 out]
        n1031 = local read "AO2"() -> (w1589:dbl)
        n1032 = local read "AO1"() -> (w1586:dbl)
        n1033 = Multiply(x=w1586, y=w1590) -> (x*y=w1585:dbl)
        n1034 = Multiply(x=w1589, y=w1590) -> (x*y=w1588:dbl)
        n1035 = Divide(x=w1585, y=w1591) -> (x/y=w1584:dbl)
        n1036 = Divide(x=w1588, y=w1591) -> (x/y=w1587:dbl)
        n1037 = To Word Integer(number=w1584) -> (16bit integer=w1592:i16)
        n1038 = To Word Integer(number=w1587) -> (16bit integer=w1593:i16)
        n1039 = xnode "Read/Write Control"("FPGA VI Reference In"=w1583, "error in"=w1582, "AO1"=w1592, "AO2"=w1593) -> ("error out"=w1581:errorcluster)  [unwired: 1 out]
      }
      event "Inject Bottom:": Value Change {
        n1040 = event-data() -> ()  [unwired: 7 out]
        n1041 = disable-structure shown="Enabled" {
          disable-tunnel: "Inject Bottom:" -> [w1595 w1635]
          frame Disabled {
            n1042 = local read "Chemyx Syringe Pump Serial Port"() -> (w1596:refnum<visa-resource-name>)
            n1043 = local read "Pump write delay (ms)"() -> (w1597:dbl)
            n1044 = case shown="True" w1595 {
              tunnel: w1597 -> [w1603 w1617]
              tunnel: w1596 -> [w1600 w1616]
              frame False {
                n1045 = flat-sequence {
                  tunnel: w1600 -> [w1604]
                  tunnel: [w1604] -> w1601
                  tunnel: w1603 -> [_]
                  tunnel: [w1607] -> w1602
                  tunnel: w1601 -> [w1607]
                  tunnel: w1602 -> [w1608]
                  tunnel: [w1608] -> w1598
                  tunnel: [w1610] -> w1599
                  tunnel: w1598 -> [w1610]
                  tunnel: w1599 -> [w1612]
                  frame #0 {
                    n1046 = call "Write to pump.vi"("string"="enter pump1", "VISA resource name"=w1604) -> ()  [unwired: 1 out]
                  }
                  frame #1 {
                    n1047 = Wait (ms)(milliseconds to wait="Pump pause delay (ms)") -> ()  [unwired: 1 out]
                  }
                  frame #2 {
                    n1048 = call "Write to pump.vi"("string"="stop", "VISA resource name"=w1608) -> ()  [unwired: 1 out]
                  }
                  frame #3 {
                    n1049 = Wait (ms)(milliseconds to wait=u32 500) -> ()  [unwired: 1 out]
                  }
                  frame #4 {
                    n1050 = call "Write to pump.vi"("string"="stop", "VISA resource name"=w1612) -> ()  [unwired: 1 out]
                  }
                }
              }
              frame True {
                n1051 = flat-sequence {
                  tunnel: w1616 -> [w1626]
                  tunnel: w1617 -> [w1621]
                  tunnel: w1617 -> [w1628]
                  tunnel: w1616 -> [w1629]
                  tunnel: [w1629] -> w1614
                  tunnel: [w1631] -> w1615
                  tunnel: w1614 -> [w1631]
                  tunnel: w1615 -> [w1633]
                  frame #0 {
                    n1052 = local read "All Pump Parameters"() -> (w1620:T6)
                    n1053 = Unbundle By Name(w1620) -> ("Pump 1"=w1627:T32)
                    n1054 = call "Set pump parameters.vi"("Pump write delay (ms)"=w1621, "Volume (uL)"="Ch 2 Inject Volume (uL)", "Rate (uL/h)"="Ch 1 Inject Rate (ul/h)", "Units"=4.0, "Pump #"=1.0, "Pump Parameters In"=w1627, "VISA resource name"=w1626) -> ("Pump Parameters Out"=w1619:T32)  [unwired: 3 in]
                    n1055 = Bundle By Name(cluster=w1620, "Pump 1"=w1619) -> (w1618:T6)
                    n1056 = local write "All Pump Parameters"(w1618) -> ()
                  }
                  frame #1 {
                    n1057 = Wait (ms)(milliseconds to wait=w1628) -> ()  [unwired: 1 out]
                  }
                  frame #2 {
                    n1058 = call "Write to pump.vi"("string"="start", "VISA resource name"=w1629) -> ()  [unwired: 1 out]
                  }
                  frame #3 {
                    n1059 = Wait (ms)(milliseconds to wait=u32 500) -> ()  [unwired: 1 out]
                  }
                  frame #4 {
                    n1060 = call "Write to pump.vi"("string"="start", "VISA resource name"=w1633) -> ()  [unwired: 1 out]
                  }
                }
              }
            }
          }
          frame Enabled {
            n1061 = call "hamilton_controller.vi"("Open?"=w1635, "valve"=enum16{"A", "B", "C", "D", "ALL"}."B", "action"=T20."MOVE VALVE") -> ()  [unwired: 8 in, 1 out]
          }
        }
      }
      event "Inject Top:": Value Change {
        n1062 = event-data() -> ()  [unwired: 7 out]
        n1063 = disable-structure shown="Disabled" {
          disable-tunnel: "Inject Top:" -> [_ w1679]
          frame Disabled {
            n1064 = local read "Pump write delay (ms)"() -> (w1640:dbl)
            n1065 = case shown="False" w1641 {
              tunnel: w1640 -> [w1647 w1661]
              tunnel: "Chemyx Syringe Pump Serial Port" -> [w1644 w1660]
              frame False {
                n1066 = flat-sequence {
                  tunnel: w1644 -> [w1648]
                  tunnel: [w1648] -> w1645
                  tunnel: w1647 -> [_]
                  tunnel: [w1651] -> w1646
                  tunnel: w1645 -> [w1651]
                  tunnel: w1646 -> [w1652]
                  tunnel: [w1652] -> w1642
                  tunnel: [w1654] -> w1643
                  tunnel: w1642 -> [w1654]
                  tunnel: w1643 -> [w1656]
                  frame #0 {
                    n1067 = call "Write to pump.vi"("string"="enter pump3", "VISA resource name"=w1648) -> ()  [unwired: 1 out]
                  }
                  frame #1 {
                    n1068 = local read "Pump pause delay (ms)"() -> (w1650:u32)
                    n1069 = Wait (ms)(milliseconds to wait=w1650) -> ()  [unwired: 1 out]
                  }
                  frame #2 {
                    n1070 = call "Write to pump.vi"("string"="stop", "VISA resource name"=w1652) -> ()  [unwired: 1 out]
                  }
                  frame #3 {
                    n1071 = Wait (ms)(milliseconds to wait=u32 0) -> ()  [unwired: 1 out]
                  }
                  frame #4 {
                    n1072 = call "Write to pump.vi"("string"="stop", "VISA resource name"=w1656) -> ()  [unwired: 1 out]
                  }
                }
              }
              frame True {
                n1073 = flat-sequence {
                  tunnel: w1660 -> [w1670]
                  tunnel: w1661 -> [w1665]
                  tunnel: w1661 -> [w1672]
                  tunnel: w1660 -> [w1673]
                  tunnel: [w1673] -> w1658
                  tunnel: [w1676] -> w1659
                  tunnel: w1658 -> [w1676]
                  tunnel: w1659 -> [w1677]
                  frame #0 {
                    n1074 = local read "All Pump Parameters"() -> (w1664:T6)
                    n1075 = Unbundle By Name(w1664) -> ("Pump 3"=w1671:T32)
                    n1076 = call "Set pump parameters.vi"("Pump write delay (ms)"=w1665, "Volume (uL)"="Ch 3 Inject Volume (uL)", "Rate (uL/h)"="Ch 3 Inject Rate (ul/h)", "Units"=4.0, "Pump #"=3.0, "Pump Parameters In"=w1671, "VISA resource name"=w1670) -> ("Pump Parameters Out"=w1663:T32)  [unwired: 3 in]
                    n1077 = Bundle By Name(cluster=w1664, "Pump 3"=w1663) -> (w1662:T6)
                    n1078 = local write "All Pump Parameters"(w1662) -> ()
                  }
                  frame #1 {
                    n1079 = Wait (ms)(milliseconds to wait=w1672) -> ()  [unwired: 1 out]
                  }
                  frame #2 {
                    n1080 = call "Write to pump.vi"("string"="start", "VISA resource name"=w1673) -> ()  [unwired: 1 out]
                  }
                  frame #3 {
                    n1081 = Wait (ms)(milliseconds to wait=u32 500) -> ()  [unwired: 1 out]
                  }
                  frame #4 {
                    n1082 = call "Write to pump.vi"("string"="start", "VISA resource name"=w1677) -> ()  [unwired: 1 out]
                  }
                }
              }
            }
          }
          frame Enabled {
            n1083 = call "hamilton_controller.vi"("Open?"=w1679, "valve"=enum16{"A", "B", "C", "D", "ALL"}."A", "action"=T20."MOVE VALVE") -> ()  [unwired: 8 in, 1 out]
          }
        }
      }
      event "Inject Valve B": Value Change {
        n1084 = event-data() -> ()  [unwired: 7 out]
        n1085 = disable-structure shown="Enabled" {
          disable-tunnel: "Inject Valve B" -> [w1683 w1703]
          frame Disabled {
            n1086 = local read "Pump write delay (ms)"() -> (w1685:dbl)
